vi "Solenoid.vi"(8 "Error In":errorcluster, 10 "TEMP,FLOW":enum8{"ENERGIZE", "DE-ENERGIZE", ""}(ring), 11 "VISA session":refnum<visa-resource-name>="MW100") -> (0 "Error Out":errorcluster, 3 "dup VISA session":refnum<visa-resource-name>)   [LabVIEW 2009]
panel:
  in  "Relay Range (001)":string="041"
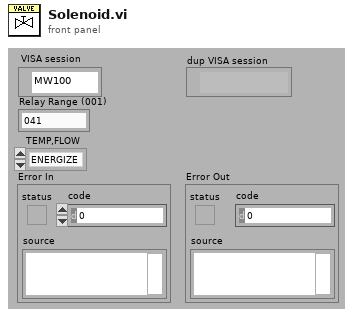
[diagram p1: front panel]
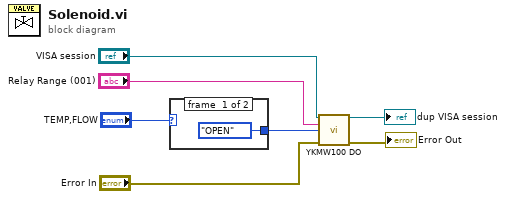
[diagram p0: block diagram]
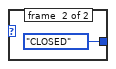
[diagram p2: hidden frame]
diagram:
  n1 = case shown="\"DE-ENERGIZE\"" "TEMP,FLOW" {
    tunnel: [enum8{"CLOSED", "OPEN"}."OPEN" ("Relay Status (0:CLOSED)") enum8{"CLOSED", "OPEN"}."CLOSED" ("Relay Status (0:CLOSED)")] -> w1
    frame #0 {
    }
    frame #1 {
    }
  }
  n2 = call "YKMW100 DO.vi"("VISA session"="VISA session", "P1 - Channel"="Relay Range (001)", "Relay Status (0:CLOSED)"=w1, "error in (no error)"="Error In") -> ("dup VISA session"=→"dup VISA session":refnum<visa-resource-name>, "error out"=→"Error Out":errorcluster)  [unwired: 10 in]
